vi "tSU_STA.vi"(0 "waveform":waveform(dbl), 2 "Index":dbl[](array[numeric]), 3 "VDDA":dbl=2.5) -> (11 "Data Binary":bool[](array[boolean])=[TRUE, TRUE, TRUE, TRUE, TRUE, FALSE, FALSE, TRUE, TRUE, TRUE, FALSE, TRUE], 12 "Data":u32=2975 format="%.0x", 13 "Data ACK":bool, 14 "Address":u32=2975 format="%.0x", 15 "Address ACK":bool, 16 "Address Binary":bool[](array[boolean])=[TRUE, TRUE, TRUE, TRUE, TRUE, FALSE, FALSE, TRUE, TRUE, TRUE, FALSE, TRUE], 17 "Reg Address":u32=2975 format="%.0x", 18 "Reg Address ACK":bool, 19 "Reg Address  Binary":bool[](array[boolean])=[TRUE, TRUE, TRUE, TRUE, TRUE, FALSE, FALSE, TRUE, TRUE, TRUE, FALSE, TRUE])   [LabVIEW 2019]
panel:
  out "Data 3":dbl[](array[numeric])
  out "Reg Address":dbl[](array[numeric])
  out "Address 2":dbl[](array[numeric])
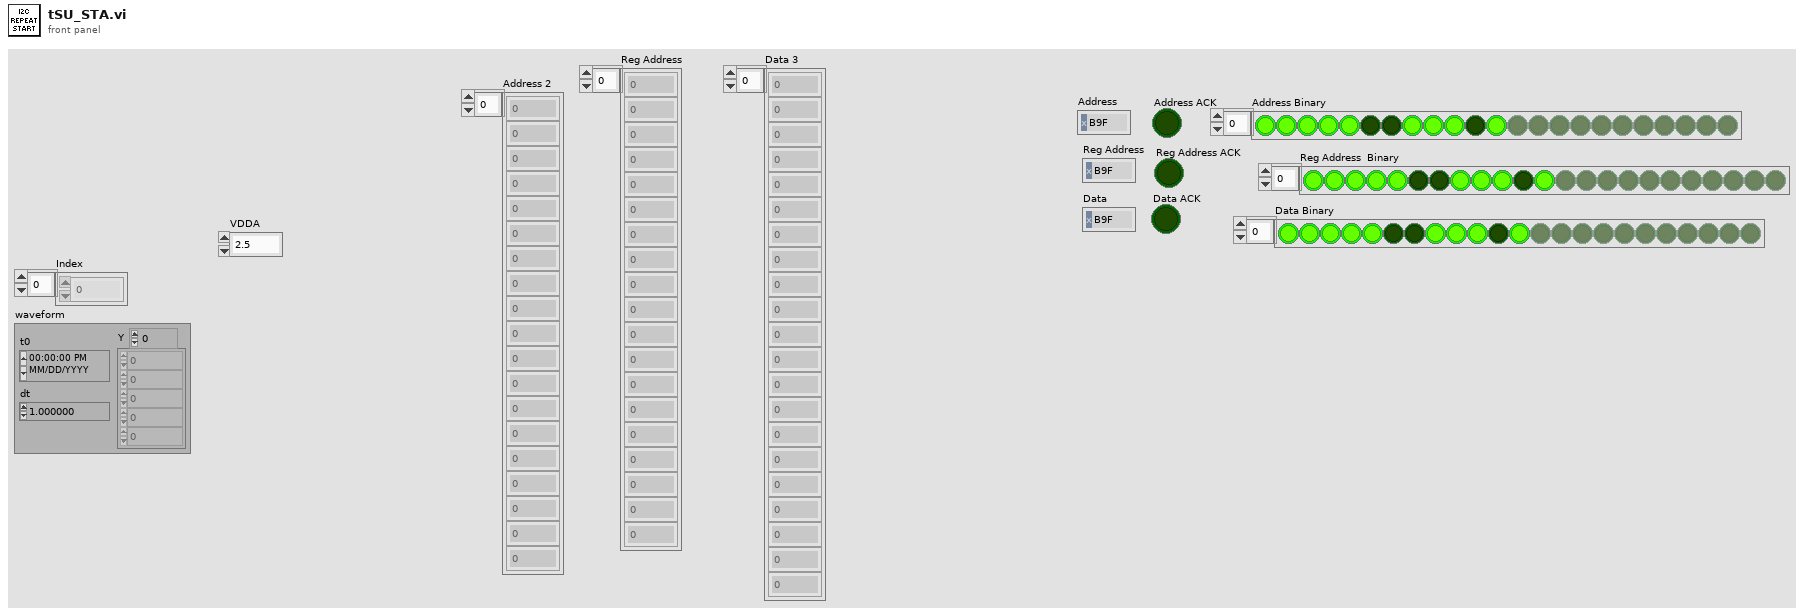
[diagram p1: front panel]
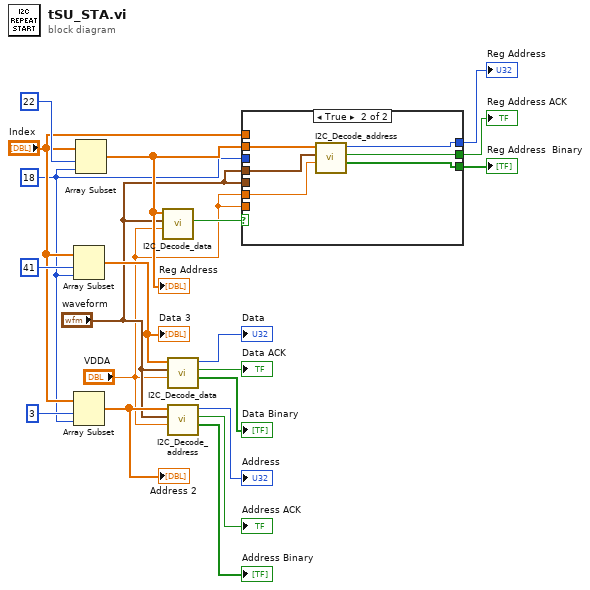
[diagram p0: block diagram]
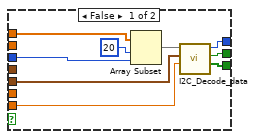
[diagram p2: hidden frame]
diagram:
  w3 = 18 ("length")
  n1 = Array Subset(array="Index", index=41, length=w3) -> (w10:dbl[])
  "Data 3" <- w10
  n2 = Array Subset(array="Index", index=3, length=w3) -> (w17:dbl[])
  "Address 2" <- w17
  n3 = Array Subset(array="Index", index=22, length=w3) -> (w8:dbl[])
  "Reg Address" <- w8
  n4 = call "I2C_Decode_data.vi"("VDDA 3"="VDDA", "waveform"="waveform", "Index"=w8) -> ("Data ACK"=w9:bool)  [unwired: 6 in, 2 out]
  n5 = call "I2C_Decode_data.vi"("VDDA 3"="VDDA", "waveform"="waveform", "Index"=w10) -> ("Data Binary"=→"Data Binary":bool[], "Data ACK"=→"Data ACK":bool, "Data"=→"Data":u32)  [unwired: 6 in]
  n6 = call "I2C_Decode_address.vi"("VDDA"="VDDA", "waveform"="waveform", "Index"=w17) -> ("Address Binary"=→"Address Binary":bool[], "Address ACK"=→"Address ACK":bool, "Address"=→"Address":u32)  [unwired: 6 in]
  n7 = case shown="True" w9 {
    tunnel: w8 -> [_ w35]
    tunnel: "waveform" -> [_ w34]
    tunnel: [w23 w33] -> w7
    tunnel: [w21 w32] -> w6
    tunnel: [w22 w31] -> w5
    tunnel: "Index" -> [w29 _]
    tunnel: w3 -> [w27 _]
    tunnel: "waveform" -> [w25 _]
    tunnel: "VDDA" -> [w24 _]
    tunnel: "VDDA" -> [_ w30]
    frame False {
      n8 = Array Subset(array=w29, index=20, length=w27) -> (w26:dbl[])
      n9 = call "I2C_Decode_data.vi"("VDDA 3"=w24, "waveform"=w25, "Index"=w26) -> ("Data Binary"=w21:bool[], "Data ACK"=w22:bool, "Data"=w23:u32)  [unwired: 6 in]
    }
    frame True {
      n10 = call "I2C_Decode_address.vi"("VDDA"=w30, "waveform"=w34, "Index"=w35) -> ("Address Binary"=w32:bool[], "Address ACK"=w31:bool, "Address"=w33:u32)  [unwired: 6 in]
    }
  }
  "Reg Address  Binary" <- w6
  "Reg Address ACK" <- w5
  "Reg Address" <- w7
